vi "interpolFilter.vi"(0 "reference in":refnum<class "subject.lvclass">, 5 "error in (no error)":errorcluster) -> (14 "reference out":refnum<class "subject.lvclass">, 19 "error out":errorcluster)   [LabVIEW 2015, in "subject.lvclass"]
uses:
  subject.lvclass
  <vilib>/gmath/NI_Gmath.lvlib
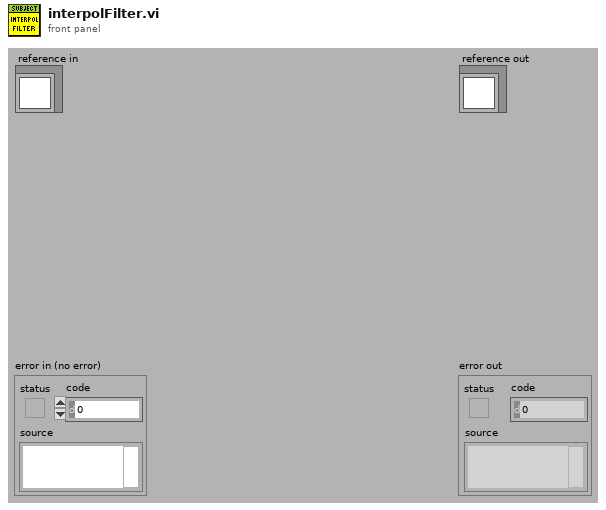
[diagram p1: front panel]
types:
  T1 = typedef "subject.lvclass/ObjectAttributesRef.ctl" = refnum<data-value>
  T2 = typedef "subject.lvclass/ObjectAttributes.ctl" = cluster{"MyAttribute":dbl, "data":cluster{"Ve_warm":dbl[], "time_warm":dbl[], "name":string, "phase":dbl[], "VCO2":dbl[], "VO2":dbl[], "PetCO2":dbl[], "RQ":dbl[], "HR":dbl[], "Ve_warm_inter":dbl[], "time_warm_inter":dbl[], "Ve_exer":dbl[], "time_exer":dbl[], "Ve_exer_inter":dbl[], "time_exer_inter":dbl[], "Ve":dbl[], "time":dbl[], "Ve_exer_inter_filtered":dbl[], "Ve_warm_inter_filtered":dbl[]}, "results_5l":cluster{"EOV":bool, "osci_amplitude":dbl[], "osci_width":dbl[], "peak_location":dbl[], "threshold":dbl, "width":i32}, "results_15percent":cluster{"EOV":bool, "osci_amplitude":dbl[], "osci_width":dbl[], "peak_location":dbl[], "threshold":dbl, "width":i32}, "supportData":cluster{"peaksAmplitude":dbl[], "iPeaksLocation":dbl[], "valesAmplitude":dbl[], "iValesLocation":dbl[], "threshold":dbl, "meanAmpl_warm":i32, "#_peaks":i32, "width":i32}, "results_user_selection":cluster{"EOV":bool, "osci_amplitude":dbl[], "osci_width":dbl[], "peak_location":dbl[], "threshold":dbl, "width":i32}, "results_warm_up":cluster{"EOV":bool, "osci_amplitude":dbl[], "osci_width":dbl[], "peak_location":dbl[], "threshold":dbl, "width":i32}}
  T3 = cluster{"Ve_warm":dbl[], "time_warm":dbl[], "name":string, "phase":dbl[], "VCO2":dbl[], "VO2":dbl[], "PetCO2":dbl[], "RQ":dbl[], "HR":dbl[], "Ve_warm_inter":dbl[], "time_warm_inter":dbl[], "Ve_exer":dbl[], "time_exer":dbl[], "Ve_exer_inter":dbl[], "time_exer_inter":dbl[], "Ve":dbl[], "time":dbl[], "Ve_exer_inter_filtered":dbl[], "Ve_warm_inter_filtered":dbl[]}
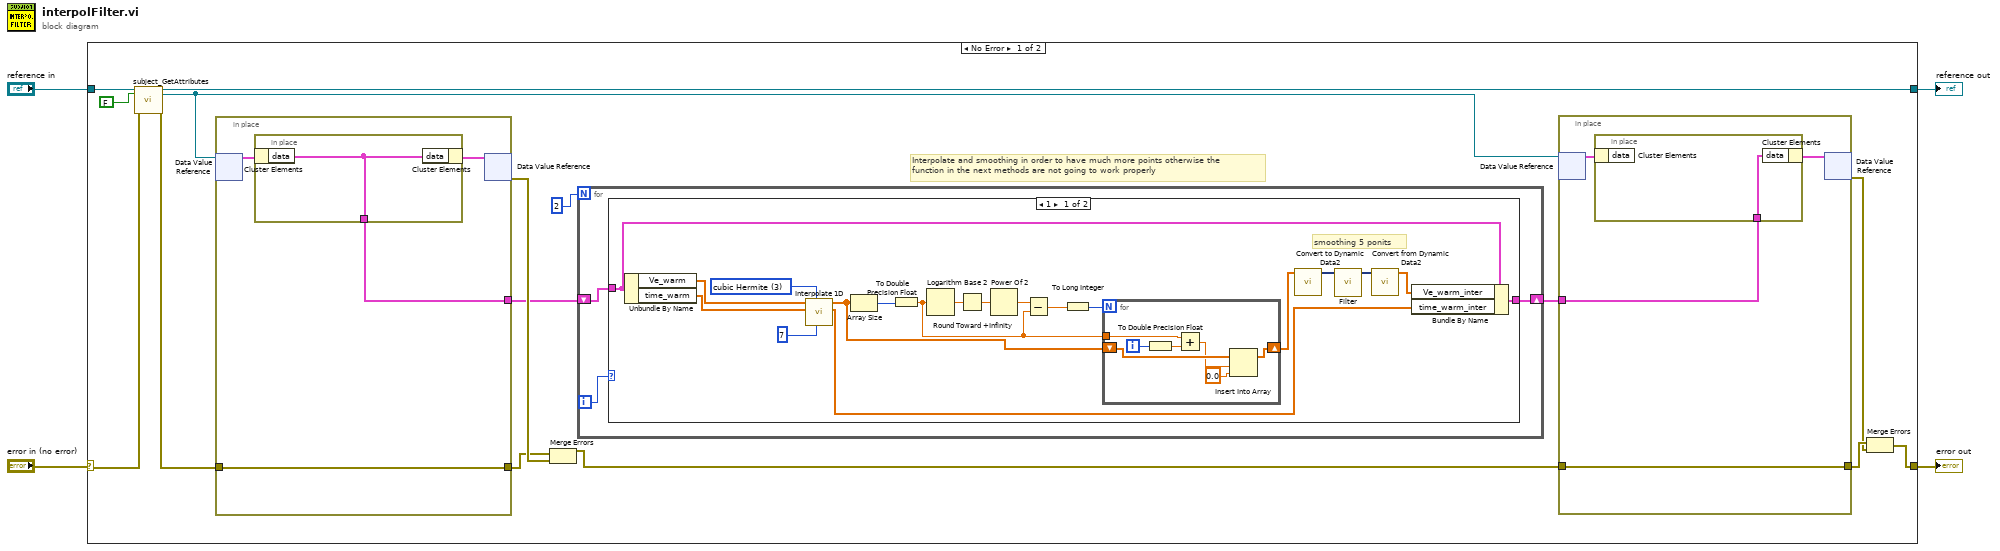
[diagram p0: block diagram]
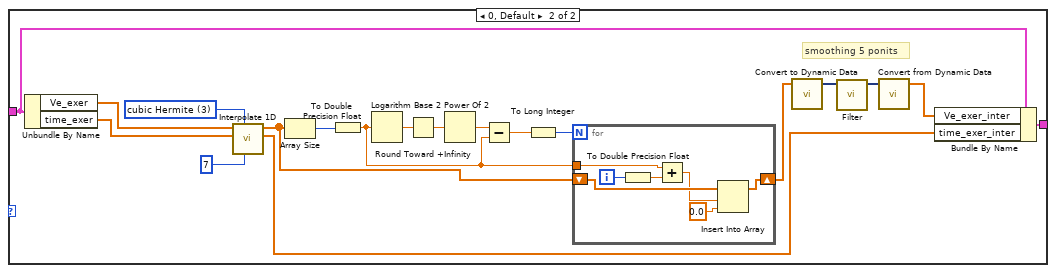
[diagram p2: hidden frame]
diagram:
  n1 = case shown="No Error" "error in (no error)" {
    selector: "error in (no error)" -> [w15 w86]
    tunnel: [w8 w86] -> w3
    tunnel: [w13 w85] -> w1
    tunnel: "reference in" -> [w17 w85]
    frame No Error {
      # "Interpolate and smoothing in order to have much more points otherwise the\nfunction in the next methods are not going to work properly"
      n2 = call "subject_GetAttributes.vi"("reference in"=w17, "return data? (T)"=FALSE, "error in (no error)"=w15) -> ("reference out"=w13:refnum<class "subject.lvclass">, "attributes ref"=w7:T1, "error out"=w14:errorcluster)  [unwired: 13 in, 1 out]
      n3 = in-place {
        in-place-border: w14 -> [w81]
        in-place-border: [w81] -> w18
        in-place-border: [w80] -> w12
        n4 = in-place-dvr #1(w7) -> (w82:T2)  [unwired: 1 out]
        n5 = in-place {
          in-place-border: [w84] -> w80
          n6 = in-place-cluster #2(w82) -> ("data"=w84:T3)
          n7 = in-place-cluster #2("data"=w84) -> (w83:T2)
        }
        n8 = in-place-dvr #1(w83) -> (w19:errorcluster)  [unwired: 1 out]
      }
      n9 = Merge Errors(w18, w19) -> (w11:errorcluster)
      n10 = for {
        N: 2 -> [_]
        shift-right: [w21] -> w5
        shift-left: w12 -> [w22]
        i -> [w20]
        n11 = case shown="1" w20 {
          tunnel: w22 -> [w23 w49]
          tunnel: [w28 w54] -> w21
          frame 1 {
            w38 = 3 items=["nearest", "linear", "spline", "cubic Hermite", "Lagrange"] ("method")
            # "smoothing 5 ponits"
            n12 = Unbundle By Name(w23) -> ("Ve_warm"=w31:dbl[], "time_warm"=w30:dbl[])
            n13 = call <vilib>:"Interpolate 1D.vi"("ntimes"=7, "method"=w38, "X"=w30, "Y"=w31) -> ("xi used"=w29:dbl[], "yi"=w40:dbl[])  [unwired: 5 in, 1 out]
            n14 = Array Size(array=w40) -> (size(s)=w41:i32)
            n15 = To Double Precision Float(number=w41) -> (double precision float=w37:dbl)
            n16 = Logarithm Base 2(1:w37) -> (0:w32:dbl)
            n17 = Round Toward +Infinity(x=w32) -> (ceil(x): smallest int >= x=w33:dbl)
            n18 = Power Of 2(x=w33) -> (2^x=w34:dbl)
            n19 = Subtract(x=w34, y=w37) -> (x-y=w35:dbl)
            n20 = To Long Integer(number=w35) -> (32bit integer=w36:i32)
            n21 = for {
              N: w36 -> [_]
              shift-right: [w46] -> w25
              shift-left: w40 -> [w48]
              tunnel: w37 -> [w45]
              i -> [w44]
              n22 = To Double Precision Float(number=w44) -> (double precision float=w43:dbl)
              n23 = Add(x=w45, y=w43) -> (x+y=w42:dbl)
              n24 = Insert Into Array(array=w48, index=w42, new element=0.0 ("new element/subarray")) -> (w46:dbl[])
            }
            n25 = call "Convert to Dynamic Data2"("Array"=w25) -> ("Dynamic Data Type"=w27:dynamicdata)  [unwired: 3 in]
            n26 = call "Filter"("Signal"=w27) -> ("Filtered Signal"=w26:dynamicdata)  [unwired: 9 in, 1 out]
            n27 = call "Convert from Dynamic Data2"("Dynamic Data Type"=w26) -> ("Array"=w24:dbl[])  [unwired: 3 in]
            n28 = Bundle By Name(cluster=w23, "Ve_warm_inter"=w24, "time_warm_inter"=w29) -> (w28:T3)
          }
          frame 0, Default {
            w64 = 3 items=["nearest", "linear", "spline", "cubic Hermite", "Lagrange"] ("method")
            # "smoothing 5 ponits"
            n29 = Unbundle By Name(w49) -> ("Ve_exer"=w57:dbl[], "time_exer"=w56:dbl[])
            n30 = call <vilib>:"Interpolate 1D.vi"("ntimes"=7, "method"=w64, "X"=w56, "Y"=w57) -> ("xi used"=w55:dbl[], "yi"=w66:dbl[])  [unwired: 5 in, 1 out]
            n31 = Array Size(array=w66) -> (size(s)=w67:i32)
            n32 = To Double Precision Float(number=w67) -> (double precision float=w63:dbl)
            n33 = Logarithm Base 2(1:w63) -> (0:w58:dbl)
            n34 = Round Toward +Infinity(x=w58) -> (ceil(x): smallest int >= x=w59:dbl)
            n35 = Power Of 2(x=w59) -> (2^x=w60:dbl)
            n36 = Subtract(x=w60, y=w63) -> (x-y=w61:dbl)
            n37 = To Long Integer(number=w61) -> (32bit integer=w62:i32)
            n38 = for {
              N: w62 -> [_]
              shift-right: [w72] -> w51
              shift-left: w66 -> [w74]
              tunnel: w63 -> [w71]
              i -> [w70]
              n39 = To Double Precision Float(number=w70) -> (double precision float=w69:dbl)
              n40 = Add(x=w71, y=w69) -> (x+y=w68:dbl)
              n41 = Insert Into Array(array=w74, index=w68, new element=0.0 ("new element/subarray")) -> (w72:dbl[])
            }
            n42 = call "Convert to Dynamic Data"("Array"=w51) -> ("Dynamic Data Type"=w53:dynamicdata)  [unwired: 3 in]
            n43 = call "Filter"("Signal"=w53) -> ("Filtered Signal"=w52:dynamicdata)  [unwired: 9 in, 1 out]
            n44 = call "Convert from Dynamic Data"("Dynamic Data Type"=w52) -> ("Array"=w50:dbl[])  [unwired: 3 in]
            n45 = Bundle By Name(cluster=w49, "Ve_exer_inter"=w50, "time_exer_inter"=w55) -> (w54:T3)
          }
        }
      }
      n46 = in-place {
        in-place-border: w11 -> [w76]
        in-place-border: [w76] -> w10
        in-place-border: w5 -> [w75]
        n47 = in-place-dvr #3(w7) -> (w77:T2)  [unwired: 1 out]
        n48 = in-place {
          in-place-border: w75 -> [w79]
          n49 = in-place-cluster #4(w77) -> ()  [unwired: 1 out]
          n50 = in-place-cluster #4("data"=w79) -> (w78:T2)
        }
        n51 = in-place-dvr #3(w78) -> (w9:errorcluster)  [unwired: 1 out]
      }
      n52 = Merge Errors(w10, w9) -> (w8:errorcluster)
    }
    frame Error {
    }
  }
  "error out" <- w3
  "reference out" <- w1
